vi "Tank Level (SubVI).vi"(10 "Fuel Tank Input":dbl, 11 "Ox Tank  Input":dbl) -> (2 "Fuel Tank Output":dbl, 3 "Ox Tank Output":dbl)   [LabVIEW 2020]
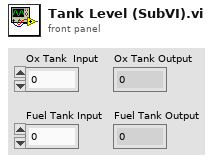
[diagram p1: front panel]
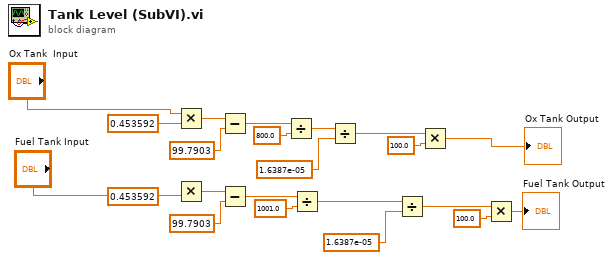
[diagram p0: block diagram]
diagram:
  n1 = Multiply(x="Ox Tank  Input", y=0.453592) -> (x*y=w12:dbl)
  n2 = Multiply(x="Fuel Tank Input", y=0.453592) -> (x*y=w3:dbl)
  n3 = Subtract(x=w12, y=99.7903) -> (x-y=w13:dbl)
  n4 = Subtract(x=w3, y=99.7903) -> (x-y=w4:dbl)
  n5 = Divide(x=w13, y=800.0) -> (x/y=w15:dbl)
  n6 = Divide(x=w4, y=1001.0) -> (x/y=w6:dbl)
  n7 = Divide(x=w15, y=1.6387e-05) -> (x/y=w17:dbl)
  n8 = Divide(x=w6, y=1.6387e-05) -> (x/y=w8:dbl)
  n9 = Multiply(x=w17, y=100.0) -> (x*y=→"Ox Tank Output":dbl)
  n10 = Multiply(x=w8, y=100.0) -> (x*y=→"Fuel Tank Output":dbl)
